vi "Actor Core.vi"(8 "error in":errorcluster, 11 "MC-ExternClient in":refnum<class "MC-ExternClient.lvclass">) -> (0 "error out":errorcluster, 3 "Actor out":refnum<class "Actor.lvclass">)   [LabVIEW 2020, in "MC-ExternClient.lvlib" / "MC-ExternClient.lvclass"]
doc: "(<B>Filename</B>: Actor Framework.lvlib:Actor.lvclass:Actor Core.vi)\n\nReceives messages to the actor, reacts to them, and initiates any error handling that may shut the actor down.\n\nDescendant classes may override this VI to append parallel tasks for the actor to complete while it handles messages. Overrides use the Call Parent Class Method node."
uses:
  MC-ExternClient.lvclass
  C:/Program Files (x86)/National Instruments/LabVIEW 2020/vi.lib/ActorFramework/Actor/Actor.lvclass
  <vilib>/ActorFramework/Actor/Actor.lvclass
  <vilib>/ActorFramework/Actor/Actor.lvclass/Actor.ctl
  <vilib>/ActorFramework/Message Enqueuer/Message Enqueuer.lvclass/Message Enqueuer.ctl
  MC-ExternClient.lvclass/MC-ExternClient.ctl
  MailboxManager/MailboxManager Messages/AddListenerMailbox Msg/AddListenerMailbox Msg.lvclass/AddListenerMailbox Msg.ctl
  MC-ExternClient Messages/SendMsgByStrType Msg/SendMsgByStrType Msg.lvclass/SendMsgByStrType Msg.ctl
  <vilib>/ActorFramework/Message Enqueuer/Init from Existing Queue.vi
  <vilib>/ActorFramework/Message Enqueuer/Enqueue.vi
  MailboxManager/MailboxManager Messages/AddListenerMailbox Msg/AddListenerMailbox Msg.lvclass
  C:/Program Files (x86)/National Instruments/LabVIEW 2020/vi.lib/ActorFramework/Message/Message.lvclass
  MC-ExternClient Messages/SendMsgByStrType Msg/SendMsgByStrType Msg.lvclass
  <vilib>/ActorFramework/Message Priority Queue/Priority Enqueue.vi
  <vilib>/ActorFramework/Message Enqueuer/Message Enqueuer.lvclass
  MailboxClient/MailboxClient/MailboxClient.lvclass
  C:/Users/taylo/Projects/LabVIEW/ActorMailbox/MailboxClient/MailboxClient/MailboxClient.lvclass
  C:/Users/taylo/Projects/LabVIEW/ActorMailbox/MailboxClientInterface/MailboxClientInterface.lvclass
  C:/Users/taylo/Projects/LabVIEW/ActorMailbox/Example/ExternClient/MC-ExternClient/MC-ExternClient/MC-ExternClient.lvclass
panel:
  in  "Data":string
  in  "Send":bool
  in  "Listbox":i32(listbox)
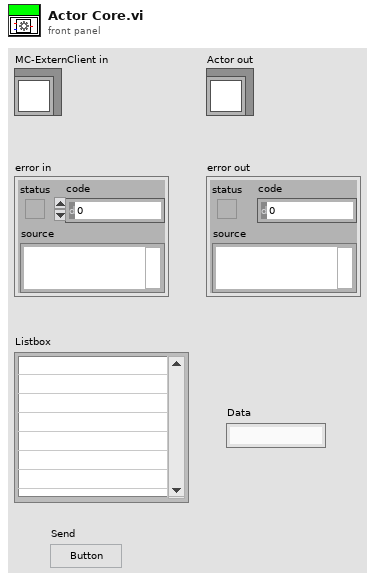
[diagram p1: front panel]
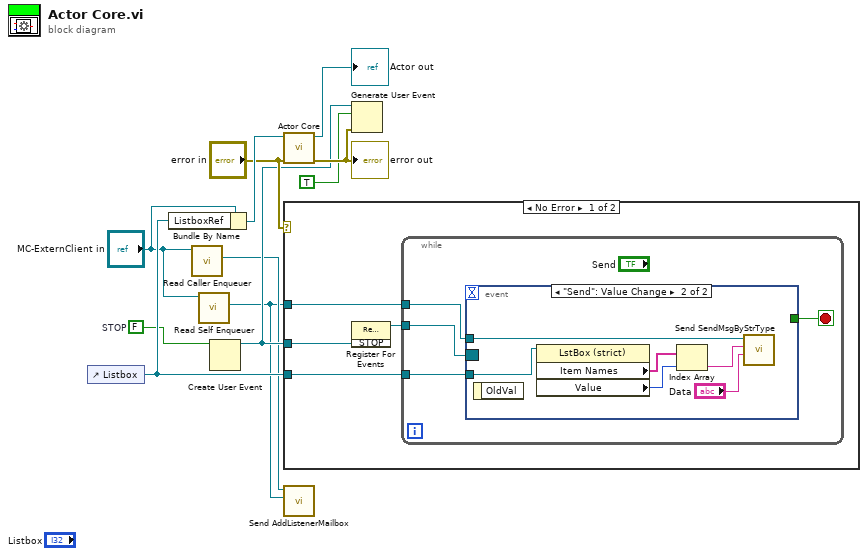
[diagram p0: block diagram]
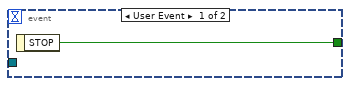
[diagram p2: hidden frame]
diagram:
  w5 = FALSE  # STOP
  n1 = control-ref of="Listbox"() -> (w8:refnum<vi>)
  n2 = Bundle By Name(cluster="MC-ExternClient in", "ListboxRef"=w8) -> (w9:refnum<class "MC-ExternClient.lvclass">)
  n3 = call <vilib>:"Read Caller Enqueuer.vi"("Actor"="MC-ExternClient in") -> ("Caller Enqueuer"=w2:refnum<class "Message Enqueuer.lvclass">)  [unwired: 10 in]
  n4 = call <vilib>:"Read Self Enqueuer.vi"("Actor"="MC-ExternClient in") -> ("Self Enqueuer"=w1:refnum<class "Message Enqueuer.lvclass">)  [unwired: 10 in]
  n5 = Create User Event(user event datatype=w5) -> (user event=w4:refnum<user-event>)  [unwired: 1 in, 1 out]
  n6 = call-parent "Actor Core.vi"("error in"="error in", "Actor in"=w9) -> ("error out"=w10:errorcluster, "Actor out"=→"Actor out":refnum<class "Actor.lvclass">)  [unwired: 8 in]
  "error out" <- w10
  n7 = case shown="No Error" "error in" {
    tunnel: w8 -> [w14 _]
    tunnel: w4 -> [w13 _]
    tunnel: w1 -> [w12 _]
    frame No Error {
      n8 = register-events(w13) -> (reference out=w15:refnum<event-registration>)  [unwired: 2 in, 1 out]
      n9 = while {
        tunnel: w15 -> [w19]
        tunnel: w14 -> [w17]
        tunnel: w12 -> [w16]
        stop <- w18 stop-if-true
        n10 = event shown="[1] \"Send\": Value Change" {
          selector: w19 -> [_ _]
          dyn-events: _ -> [_ _]
          timeout: _ -> [_ _]
          tunnel: [w20 _] -> w18
          tunnel: w17 -> [_ w26]
          tunnel: w16 -> [_ w23]
          event User Event {
            n11 = event-data() -> ("STOP"=w20:bool)  [unwired: 1 in]
          }
          event "Send": Value Change {
            n12 = event-data() -> ()  [unwired: 1 in, 1 out]
            n13 = property class="LstBox (strict)"(reference=w26) -> ("Item Names"=w24:string[], "Value"=w25:i32)  [unwired: 1 in, 2 out]
            n14 = Index Array(array=w24, index=w25) -> (element=w22:string)
            n15 = call "Send SendMsgByStrType.vi"("Data"="Data", "MSG"=w22, "Message Enqueuer"=w23) -> ()  [unwired: 7 in, 2 out]
          }
        }
      }
    }
    frame Error {
    }
  }
  n16 = call "Send AddListenerMailbox.vi"("Message Enqueuer 2"=w1, "Message Enqueuer"=w2) -> ()  [unwired: 8 in, 2 out]
  n17 = Generate User Event(user event=w4, event data cluster=TRUE ("event data"), error in=w10) -> ()  [unwired: 1 in, 2 out]
